vi "scope_BlockAcquisition.vi"() -> ()   [LabVIEW 2011]
panel:
  out "Tau vs. T":dbl(graph)
  out "Waveform Graph":dbl[](graph)
  in  "stop":bool
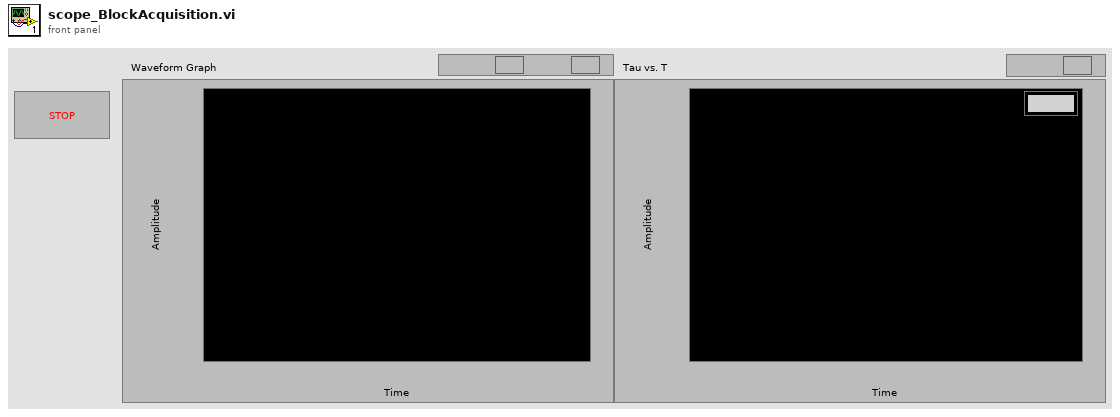
[diagram p1: front panel]
types:
  T1 = cluster{i32, "Sample Internal":sgl, "Data (Volts)":dbl[]}
  T2 = cluster{"Driver Version":string, "USB Version":string, "Hardware":string, "Variant":string, "Batch and Serial":string, "Cal Date":string, "Kernel Version":string, "Digital HW Version":string, "Analogue HW Version":string, "Firmware 1":string, "Firmware 2":string, "MSO":bool, "Number of Channels":i16}
  T3 = cluster{"preTriggerSamples":u32, "postTriggerSamples":u32, "timebase":u32, "Down-Sample Mode":i32, "Down Sample Ratio":u32, "Oversample":i16}
  T4 = cluster{"Enabled":bool, "Coupling":i16, "Range":u16, "Analogue Offset":sgl}
  T5 = cluster{"Trigger Enabled":bool, "Trigger Source":enum16{"Channel A", "Channel B", "Channel C", "Channel D", "Ext."}, "Trigger Threshold (Volts)":dbl, "Trigger Direction":u16, "Trigger Delay (samples)":u32, "Auto Trigger Time (ms)":i16}
  T6 = cluster{"Sample Frequency":sgl, "Sample Internal":sgl, "Max Samples Available":i32, "Number of Samples":u32, "Total Capture Time (sec) ":sgl, "Max Total Capture Time Available (sec)":sgl}
  T7 = cluster{"Channel D Buffer":i16[], "Channel C Buffer":i16[], "Channel B Buffer":i16[], "Channel A Buffer":i16[], "Port 0  Buffer ":i16[], "Port 1 Buffer ":i16[]}
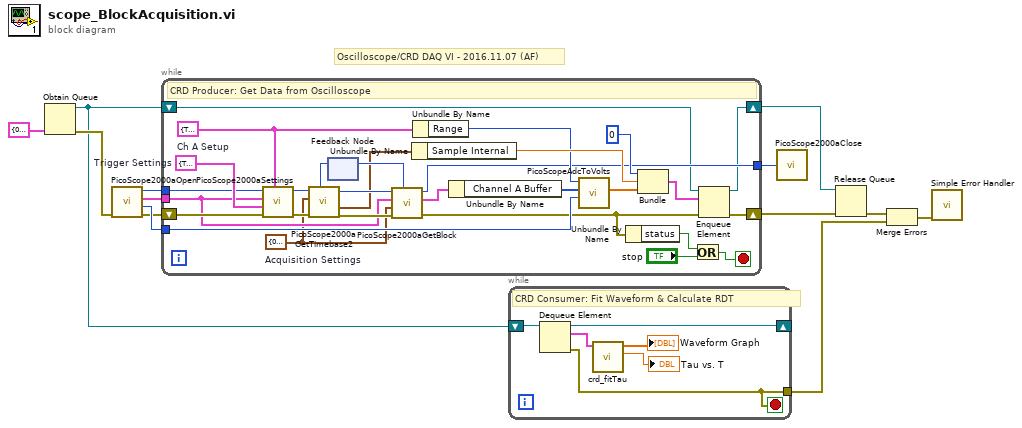
[diagram p0: block diagram]
diagram:
  # "Oscilloscope/CRD DAQ VI - 2016.11.07 (AF)"
  n1 = Obtain Queue(element data type=T1 {0, "Sample Internal"=8e-09, "Data (Volts)"=array[20000 elements]} ("Channel A 2")) -> (queue out=w5:refnum<queue>, error out=w8:errorcluster)  [unwired: 4 in, 1 out]
  n2 = call "PicoScope2000aOpen.vi"("error in (no error)"=w8) -> ("error out"=w12:errorcluster, "Max Adc value"=w13:i16, "Device Info"=w11:T2, "handle"=w10:i16)  [unwired: 7 in]
  n3 = while {
    tunnel: w11 -> [w25]
    tunnel: w10 -> [w34]
    tunnel: w13 -> [w32]
    tunnel: [w20] -> w4
    shift-right: [w18] -> w7
    shift-left: w5 -> [w15]
    shift-right: [w17] -> w6
    shift-left: w12 -> [w35]
    stop <- w41 stop-if-true
    w19 = T3 {"preTriggerSamples"=0, "postTriggerSamples"=20000, "timebase"=2, "Down-Sample Mode"=0, "Down Sample Ratio"=1, "Oversample"=1}  # Acquisition Settings
    w37 = T4 {"Enabled"=TRUE, "Coupling"=0, "Range"=1, "Analogue Offset"=0.0}  # Ch A Setup
    w36 = T5 {"Trigger Enabled"=TRUE, "Trigger Source"=enum."Channel A", "Trigger Threshold (Volts)"=0.007, "Trigger Direction"=2, "Trigger Delay (samples)"=0, "Auto Trigger Time (ms)"=1000}  # Trigger Settings
    # "CRD Producer: Get Data from Oscilloscope"
    n4 = call "PicoScope2000aSettings.vi"("Channel A Settings"=w37, "error in"=w35, "Trigger Settings"=w36, "Device Info"=w25, "handle in"=w34) -> ("error out"=w30:errorcluster, "handle out"=w31:i16)  [unwired: 5 in]
    n5 = feedback #1() -> (w28:u32)  [unwired: 1 in]
    n6 = call "PicoScope2000aGetTimebase2.vi"("Number of Samples"=w28, "error in (no error)"=w30, "Acquisition Settings"=w19, "handle in"=w31) -> ("error out"=w27:errorcluster, "Properties Panel"=w24:T6, "handle out"=w26:i16)  [unwired: 5 in]
    n7 = call "PicoScope2000aGetBlock.vi"("error in"=w27, "Acquisition Settings"=w19, "Device Info"=w25, "handle in"=w26) -> ("error out"=w14:errorcluster, "Buffers (Max or non-aggregated)"=w23:T7, "handle out"=w20:i16, "noOfSamples"=w29:u32)  [unwired: 2 in, 2 out]
    n8 = feedback-in #1(w29) -> ()
    n9 = Unbundle By Name(w24) -> ("Sample Internal"=w38:sgl)
    n10 = Unbundle By Name(w37) -> ("Range"=w33:u16)
    n11 = Unbundle By Name(w23) -> ("Channel A Buffer"=w22:i16[])
    n12 = call "PicoScopeAdcToVolts.vi"("Max_adc"=w32, "Data"=w22, "Range Index"=w33) -> ("Data (Volts)"=w39:dbl[])  [unwired: 8 in]
    n13 = Unbundle By Name(w14) -> ("status"=w21:bool)
    n14 = Bundle(0, "Sample Internal"=w38, "Data (Volts)"=w39) -> (w16:T1)  [unwired: 1 in]
    n15 = Or(x=w21, y="stop") -> (x .or. y?=w41:bool)
    n16 = Enqueue Element(queue=w15, element=w16, error in (no error)=w14) -> (queue out=w18:refnum<queue>, error out=w17:errorcluster)  [unwired: 1 in, 1 out]
  }
  n17 = while {
    shift-right: [w47] -> _
    shift-left: w5 -> [w48]
    tunnel: [w43] -> w1
    stop <- w43 stop-if-true
    # "CRD Consumer: Fit Waveform & Calculate RDT"
    n18 = Dequeue Element(queue=w48) -> (queue out=w47:refnum<queue>, element=w46:T1, error out=w43:errorcluster)  [unwired: 2 in, 1 out]
    n19 = call "crd_fitTau.vi"("Channel A in"=w46) -> ("tau (us)"=→"Tau vs. T":dbl, "Decay"=→"Waveform Graph":dbl[])  [unwired: 9 in]
  }
  n20 = call "PicoScope2000aClose.vi"("handle"=w4) -> ()
  n21 = Release Queue(queue=w7, error in (no error)=w6) -> (error out=w2:errorcluster)  [unwired: 1 in, 2 out]
  n22 = Merge Errors(w2, w1) -> (w3:errorcluster)
  n23 = call <vilib>:"Simple Error Handler.vi"("error in (no error)"=w3) -> ()  [unwired: 4 in, 5 out]
